vi "3D Robot Scene.vi"(8 "error in (no error)":errorcluster) -> (0 "error out":errorcluster, 1 "axles":refnum<vi>[](array[refnum]), 2 "robot":refnum<vi>, 3 "scene":refnum<vi>)   [LabVIEW 2017]
uses:
  <vilib>/picture/3D Picture Control/Object/Create Object (name).vi
  Robot Parameters/Robot Parameters.vi
  <vilib>/picture/3D Picture Control/NI_3D Picture Control.lvlib
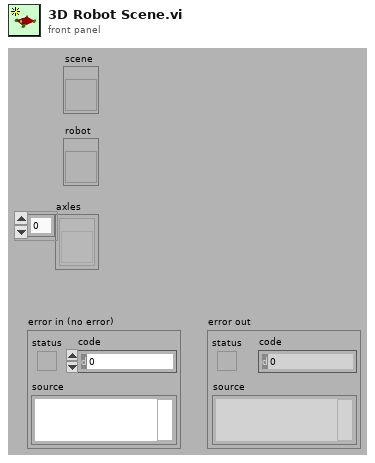
[diagram p1: front panel]
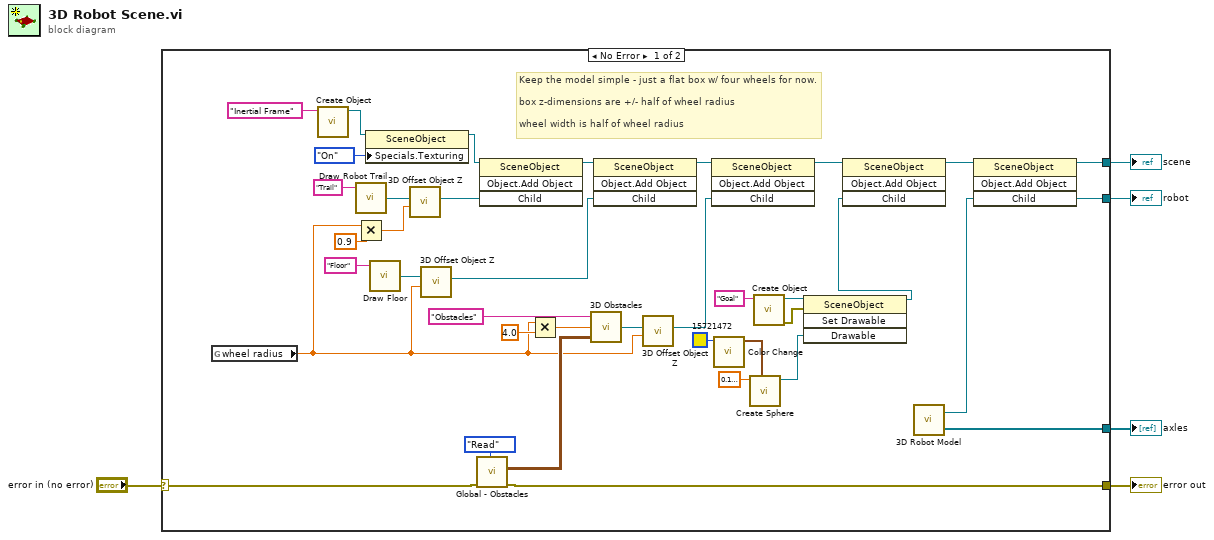
[diagram p0: block diagram]
diagram:
  n1 = case shown="No Error" "error in (no error)" {
    selector: "error in (no error)" -> [w6 w44]
    tunnel: [w43 _] -> w5
    tunnel: [w39 _] -> w4
    tunnel: [w33 _] -> w3
    tunnel: [w7 w44] -> w2
    frame No Error {
      # "Keep the model simple - just a flat box w/ four wheels for now.\n\nbox z-dimensions are +/- half of wheel radius\n\nwheel width is half of wheel radius"
      n2 = global read "Robot Parameters.vi" "wheel radius"() -> (w8:dbl)
      n3 = call-poly <vilib>:"Create Object.vi"("Name"="Inertial Frame") -> ("Scene:New Object"=w38:refnum<vi>)  [unwired: 9 in, 1 out]
      n4 = call "Draw Robot Trail.vi"("Name"="Trail") -> ("Scene:New Object"=w32:refnum<vi>)  [unwired: 4 out]
      n5 = Multiply(x=w8, y=0.9) -> (x*y=w28:dbl)
      n6 = property class="SceneObject"(reference=w38, "Specials.Texturing"=enum16{"Inherit Value", "Off", "On"}."On" ("Specials:Texturing")) -> (reference out=w34:refnum<vi>)  [unwired: 1 in, 1 out]
      n7 = call "Draw Floor.vi"("Name"="Floor") -> ("Scene.Object Out"=w30:refnum<vi>)  [unwired: 1 in, 3 out]
      n8 = call "3D Offset Object Z.vi"("Offset"=w28, "Scene:New Object"=w32) -> ("Scene.Object Out"=w31:refnum<vi>)  [unwired: 7 out]
      n9 = call "3D Offset Object Z.vi"("Offset"=w8, "Scene:New Object"=w30) -> ("Scene.Object Out"=w29:refnum<vi>)  [unwired: 7 out]
      n10 = call "Global - Obstacles.vi"("mode"=enum16{"Initialize", "Read", "Write"}."Read" ("Mode"), "error in (no error)"=w6) -> ("error out"=w7:errorcluster, "obstacles out"=w19:cluster{dbl, dbl}[][])  [unwired: 7 in, 1 out]
      n11 = invoke class="SceneObject" method="Object.Add Object"(reference=w34, "Child"=w31) -> (reference out=w35:refnum<vi>)  [unwired: 2 in, 3 out]
      n12 = Multiply(x=w8, y=4.0) -> (x*y=w25:dbl)
      n13 = call "3D Obstacles.vi"("Obstacles (n x 2 array of pts)"=w19, "Height"=w25, "Name"="Obstacles") -> ("Scene:New Object"=w23:refnum<vi>)
      n14 = invoke class="SceneObject" method="Object.Add Object"(reference=w35, "Child"=w29) -> (reference out=w22:refnum<vi>)  [unwired: 2 in, 3 out]
      n15 = call "3D Offset Object Z.vi"("Offset"=w8, "Scene:New Object"=w23) -> ("Scene.Object Out"=w21:refnum<vi>)  [unwired: 7 out]
      n16 = invoke class="SceneObject" method="Object.Add Object"(reference=w22, "Child"=w21) -> (reference out=w18:refnum<vi>)  [unwired: 2 in, 3 out]
      n17 = call <vilib>:"Color Change.vi"("Color"=u32 15721472) -> ("RGBA"=w11:cluster{"R":sgl, "G":sgl, "B":sgl, "A":sgl})  [unwired: 10 in]
      n18 = call <vilib>:"Create Sphere.vi"("Color"=w11, "Radius"=sgl 0.1) -> ("New Sphere Refnum"=w14:refnum<vi>)  [unwired: 8 in, 1 out]
      n19 = call-poly <vilib>:"Create Object.vi"("Name"="Goal") -> ("error out"=w15:errorcluster, "Scene:New Object"=w16:refnum<vi>)  [unwired: 9 in]
      n20 = invoke class="SceneObject" method="Set Drawable"(reference=w16, error in=w15, "Drawable"=w14) -> (reference out=w10:refnum<vi>)  [unwired: 1 in, 3 out]
      n21 = invoke class="SceneObject" method="Object.Add Object"(reference=w18, "Child"=w10) -> (reference out=w9:refnum<vi>)  [unwired: 2 in, 3 out]
      n22 = call "3D Robot Model.vi"() -> ("robot frame"=w41:refnum<vi>, "axles"=w43:refnum<vi>[])  [unwired: 1 in]
      n23 = invoke class="SceneObject" method="Object.Add Object"(reference=w9, "Child"=w41) -> (reference out=w33:refnum<vi>, "Child"=w39:refnum<vi>)  [unwired: 2 in, 2 out]
    }
    frame Error {
    }
  }
  "robot" <- w4
  "axles" <- w5
  "scene" <- w3
  "error out" <- w2
